vi "search hierarchy.vi"(10 "ID":string, 11 "hierarchy":T1[](array[typedef])) -> (3 "index":i32)   [LabVIEW 2013, in "NISE_CEF_TreeSerializer.lvlib"]
uses:
  NISE_CEF_TreeSerializer.lvlib
  hierarchy element.ctl
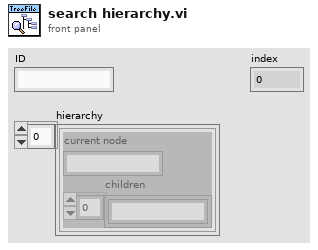
[diagram p1: front panel]
types:
  T1 = typedef "NISE_CEF_TreeSerializer.lvlib/hierarchy element.ctl" = cluster{"current node":string, "children":string[]}
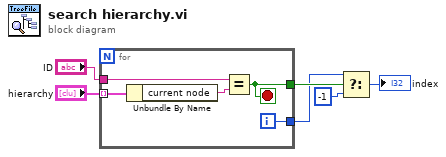
[diagram p0: block diagram]
diagram:
  n1 = for {
    tunnel: "hierarchy" -> [w11] mode=indexing
    tunnel: "ID" -> [w9]
    tunnel: [w7] -> w4
    tunnel: [w8] -> w3
    i -> [w8]
    stop <- w7 stop-if-true
    n2 = Unbundle By Name(w11) -> ("current node"=w10:string)
    n3 = Equal?(x=w9, y=w10) -> (x = y?=w7:bool)
  }
  n4 = Select(t=w3, s=w4, f=-1) -> (s? t:f=→"index":i32)
